vi "FGVfpgaAdressScanEngine.vi"(6 "zDataRateIn":u32=40000000 format="%.0p", 7 "Enum":T2=enum."Read", 8 "error in":errorcluster, 9 "ioFreqHzIn":u32=67500000 format="%.2p", 10 "FPGA.SEin":T1, 11 "voltageRange(+/-)In":dbl) -> (0 "error out":errorcluster, 1 "ioFreqHzOut":u32, 2 "FPGA.SEout":T1, 3 "voltageRange(+/-)Out":dbl, 4 "zDataRateOut":u32)   [LabVIEW 2016]
uses:
  controls/Enum.ctl
  controls/FPGAVIreferenceTypeDefScanEngine.ctl
  <vilib>/rvi/errors/niLvFpgaAdjustHostInterfaceError.vi
  <vilib>/Utility/error.llb/Error Cluster From Error Code.vi
  <vilib>/FPGAPlugInAG/USB-7856R OEM/niLvFpga_Open_USB-7856R OEM.vi
  <vilib>/rvi/interface/nirviReadWriteControl/nirviReadWriteControl.xnode
  FPGA Bitfiles/qnmController797_usbRIO_controllerFPGAmu.lvbitx
  <vilib>/rvi/interface/nirviOpenFPGA/nirviOpenFPGA.xnode
  NiFpgaLv.dll
panel:
  # "Write for the FPGA Reference has to be changed in the diagram in case need to write the adress different than RIO"
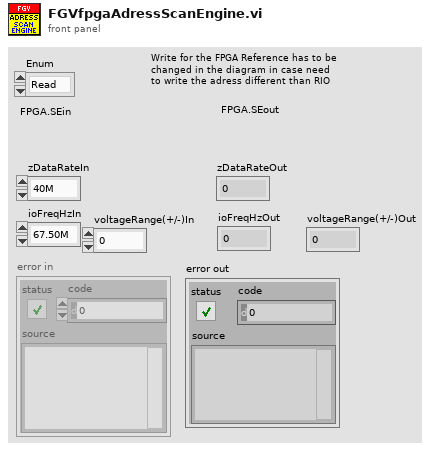
[diagram p1: front panel]
types:
  T1 = typedef "FPGAVIreferenceTypeDefScanEngine.ctl" = refnum<k20>
  T2 = typedef "Enum.ctl" = enum16{"Init", "Read", "Write"}
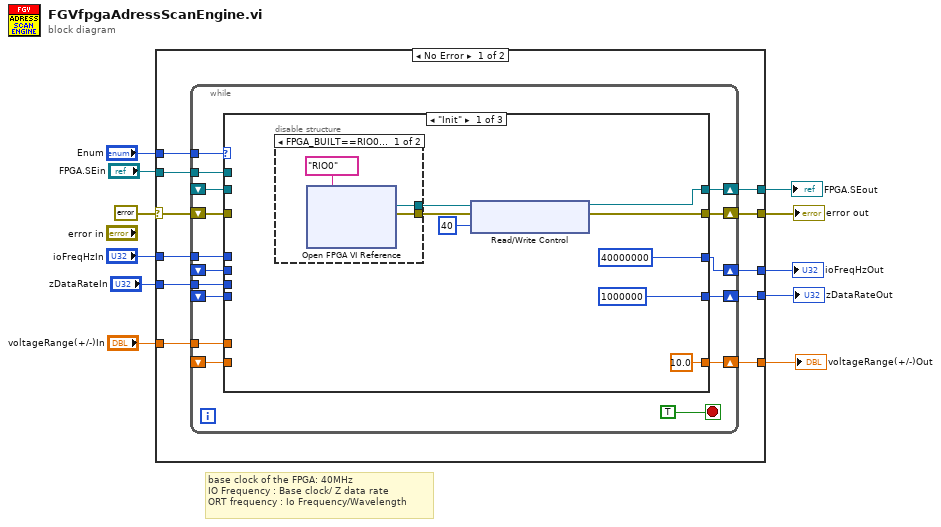
[diagram p0: block diagram]
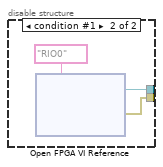
[diagram p2: hidden frame]
diagram:
  # "base clock of the FPGA: 40MHz\nIO Frequency : Base clock/ Z data rate\nORT frequency : Io Frequency/Wavelength"
  n1 = case shown="No Error" errorcluster {"status"=FALSE, "code"=0, "source"=""} ("error IO") {
    selector: errorcluster {"status"=FALSE, "code"=0, "source"=""} ("error IO") -> [w19 w67]
    tunnel: "Enum" -> [w22 _]
    tunnel: [w21 w65] -> w3
    tunnel: "FPGA.SEin" -> [w20 w65]
    tunnel: [w18 w67] -> w10
    tunnel: "ioFreqHzIn" -> [w17 w66]
    tunnel: [w16 w66] -> w8
    tunnel: "zDataRateIn" -> [w15 w64]
    tunnel: [w14 w64] -> w5
    tunnel: "voltageRange(+/-)In" -> [w13 w63]
    tunnel: [w12 w63] -> w1
    frame No Error {
      n2 = while {
        tunnel: w22 -> [w37]
        tunnel: w20 -> [w36]
        shift-right: [w35] -> w21
        shift-left: _ -> [w34]
        tunnel: w17 -> [w31]
        shift-right: [w30] -> w16
        shift-left: _ -> [w29]
        tunnel: w15 -> [w28]
        shift-right: [w27] -> w14
        shift-left: _ -> [w26]
        shift-right: [w32] -> w18
        shift-left: w19 -> [w33]
        tunnel: w13 -> [w25]
        shift-right: [w24] -> w12
        shift-left: _ -> [w23]
        stop <- TRUE stop-if-true
        n3 = case shown="\"Init\"" w37 {
          tunnel: w36 -> [_ _ _]
          tunnel: [w43 w57 w60] -> w35
          tunnel: w34 -> [_ w57 w60]
          tunnel: w33 -> [_ w56 w62]
          tunnel: [w46 w56 w62] -> w32
          tunnel: w31 -> [_ _ w61]
          tunnel: [u32 40000000 ("ioFreqHzIn") w55 w61] -> w30
          tunnel: w29 -> [_ w55 _]
          tunnel: w28 -> [_ _ w59]
          tunnel: [u32 1000000 ("zDataRate") w54 w59] -> w27
          tunnel: w26 -> [_ w54 _]
          tunnel: w25 -> [_ _ w58]
          tunnel: [10.0 ("voltageRange(+/-)In") w53 w58] -> w24
          tunnel: w23 -> [_ w53 _]
          frame "Init" {
            n4 = disable-structure shown="FPGA_BUILT==RIO0, Default" {
              disable-tunnel: [w49 w50] -> w41
              disable-tunnel: [w48 w51] -> w40
              frame condition #0 (active) {
                n5 = xnode "Open FPGA VI Reference"("resource name"=tag "RIO0") -> ("FPGA VI Reference Out"=w49:T1, "error out"=w48:errorcluster)  [unwired: 1 in]
              }
              frame condition #1 {
                n6 = xnode "Open FPGA VI Reference"("resource name"=tag "RIO0") -> ("FPGA VI Reference Out"=w50:T1, "error out"=w51:errorcluster)  [unwired: 1 in]
              }
            }
            n7 = xnode "Read/Write Control"("FPGA VI Reference In"=w41, "error in"=w40, "aio.i.slowInputRate"=u32 40 ("zDataRate")) -> ("FPGA VI Reference Out"=w43:T1, "error out"=w46:errorcluster)
          }
          frame "Read", Default {
          }
          frame "Write" {
          }
        }
      }
    }
    frame Error {
    }
  }
  "error out" <- w10
  "ioFreqHzOut" <- w8
  "zDataRateOut" <- w5
  "FPGA.SEout" <- w3
  "voltageRange(+/-)Out" <- w1
